vi "Actor Last Ack.vi"(9 "Nested Error":errorcluster, 10 "Nested Actor":refnum<class "Actor.lvclass">, 11 "Dev Actor in":refnum<class "Dev Actor.lvclass">) -> (0 "error out":errorcluster, 3 "Dev Actor out":refnum<class "Dev Actor.lvclass">)   [LabVIEW 2021, in "Dev Actor.lvlib" / "Dev Actor.lvclass"]
uses:
  Dev Actor.lvclass
  LVCAM/LVCAM/Actor/Actor.lvclass
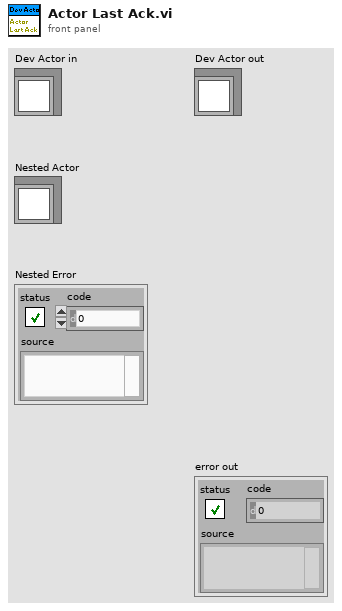
[diagram p1: front panel]
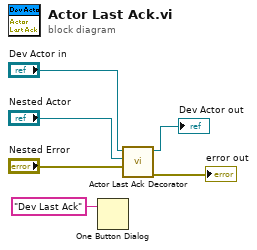
[diagram p0: block diagram]
diagram:
  n1 = One Button Dialog(message="Dev Last Ack") -> ()  [unwired: 1 in, 1 out]
  n2 = call "Actor Last Ack Decorator.vi"("Nested Error"="Nested Error", "Nested Actor"="Nested Actor", "Dev Actor in"="Dev Actor in") -> ("error out"=→"error out":errorcluster, "Dev Actor out"=→"Dev Actor out":refnum<class "Dev Actor.lvclass">)  [unwired: 7 in]
